vi "Get Boolean.vi"(1 "Name":string) -> (0 "Value":bool)   [LabVIEW 2015]
doc: "Used to retrieve boolean values for use in \"until\" subcommands."
uses:
  AppleScript Global Data.vi
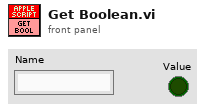
[diagram p1: front panel]
types:
  T1 = typedef "WPI_DigitalInputDevRef.ctl" = cluster{"DevStatus":errorcluster, "DIO Channel":T2}
  T2 = typedef "FPGA_DIOChannel.ctl" = enum8{"DIO 0", "DIO 1", "DIO 2", "DIO 3", "DIO 4", "DIO 5", "DIO 6", "DIO 7", "DIO 8", "DIO 9", "DIO MXP 0", "DIO MXP 1", "DIO MXP 2", "DIO MXP 3", "DIO MXP 4", "DIO MXP 5", "DIO MXP 6", "DIO MXP 7", "DIO MXP 8", "DIO MXP 9", "DIO MXP 10", "DIO MXP 11", "DIO MXP 12", "DIO MXP 13", "DIO MXP 14", "DIO MXP 15", "Invalid"}
  T3 = typedef "WPI_EncoderDevRef.ctl" = cluster{"DevStatus":errorcluster, "EncoderIndex":T4, "CounterIndex":T5, "DistancePerCount":dbl, "Decoding Type":T6}
  T4 = typedef "FPGA_EncoderIdx.ctl" = enum8{"Enc 0", "Enc 1", "Enc 2", "Enc 3", "Enc 4", "Enc 5", "Enc 6", "Enc 7", "Invalid"}
  T5 = typedef "FPGA_CounterCtrSystemIndex.ctl" = enum8{"Ctr 0", "Ctr 1", "Ctr 2", "Ctr 3", "Ctr 4", "Ctr 5", "Ctr 6", "Ctr 7", "Invalid"}
  T6 = typedef "WPI_EncoderType.ctl" = enum16{"1x", "2x", "4x"}
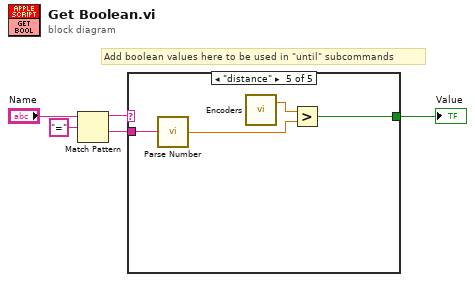
[diagram p0: block diagram]
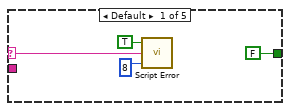
[diagram p2: hidden frame]
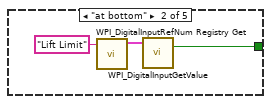
[diagram p3: hidden frame]
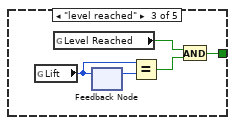
[diagram p4: hidden frame]
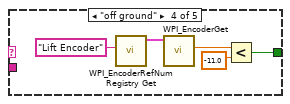
[diagram p5: hidden frame]
diagram:
  # "Add boolean values here to be used in \"until\" subcommands"
  n1 = Match Pattern(string="Name", regular expression="=") -> (before substring=w3:string, after substring=w1:string)  [unwired: 1 in, 2 out]
  n2 = case shown="\"distance\"" w3 {
    selector: w3 -> [w6 _ _ _ _]
    tunnel: [FALSE w10 w15 w18 w23] -> w5
    tunnel: w1 -> [_ _ _ _ w25]
    frame Default {
      n3 = call "Script Error.vi"("Error?"=TRUE, "Error Details"=w6, "Error Code"=8) -> ()  [unwired: 2 in, 1 out]
    }
    frame "at bottom" {
      n4 = call <vilib>:"WPI_DigitalInputRefNum Registry Get.vi"("refnum name"="Lift Limit") -> ("DigitalInputDevRef"=w11:T1)  [unwired: 9 in, 1 out]
      n5 = call <vilib>:"WPI_DigitalInputGetValue.vi"("DigitalInputDevRef"=w11) -> ("Value"=w10:bool)  [unwired: 8 in, 2 out]
    }
    frame "level reached" {
      n6 = global read "AppleScript Global Data.vi" "Lift"() -> (w17:i16)
      n7 = global read "AppleScript Global Data.vi" "Level Reached"() -> (w14:bool)
      n8 = feedback-in #1(w17) -> ()
      n9 = feedback #1() -> (w16:i16)  [unwired: 1 in]
      n10 = Equal?(x=w17, y=w16) -> (x = y?=w13:bool)
      n11 = And(x=w14, y=w13) -> (x .and. y?=w15:bool)
    }
    frame "off ground" {
      n12 = call <vilib>:"WPI_EncoderRefNum Registry Get.vi"("refnum name"="Lift Encoder") -> ("EncoderDevRef"=w22:T3)  [unwired: 9 in, 1 out]
      n13 = call <vilib>:"WPI_EncoderGet.vi"("EncoderDevRef"=w22) -> ("Distance"=w20:dbl)  [unwired: 5 in, 5 out]
      n14 = Less?(x=w20, y=-11.0) -> (x < y?=w18:bool)
    }
    frame "distance" {
      n15 = call "Parse Number.vi"("String"=w25) -> ("Number"=w24:dbl)
      n16 = call "Encoders.vi"() -> ("Avg Absolute Distance"=w26:dbl)  [unwired: 2 in, 1 out]
      n17 = Greater?(x=w26, y=w24) -> (0:w23:bool)
    }
  }
  "Value" <- w5
